vi "ErrorHandler.vi"(8 "error in (no error)":errorcluster, 11 "queue in":refnum<queue>) -> (0 "error out":errorcluster)   [LabVIEW 2024]
uses:
  Controls/MainStates.ctl
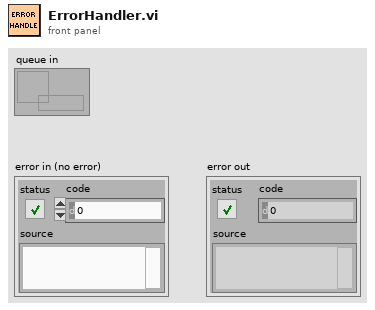
[diagram p1: front panel]
types:
  T1 = typedef "MainStates.ctl" = enum16{"Init", "Get Path", "Get Files", "Set Extension", "Check for Dups", "Clean", "Add Prefix", "Replace", "Periods", "Strip Prefix", "Commit", "Wait for Input", "Exit"}
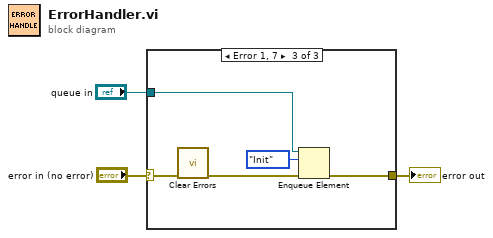
[diagram p0: block diagram]
diagram:
  n1 = case shown="Error 1, 7" "error in (no error)" {
    selector: "error in (no error)" -> [w4 w5 w10]
    tunnel: [w4 w5 w8] -> w2
    tunnel: "queue in" -> [_ _ w7]
    frame No Error {
    }
    frame Default {
    }
    frame Error {
      n2 = call <vilib>:"Clear Errors.vi"("error in (no error)"=w10) -> ("error out"=w9:errorcluster)  [unwired: 5 in, 1 out]
      n3 = Enqueue Element(queue=w7, element=MainStates."Init", error in (no error)=w9) -> (error out=w8:errorcluster)  [unwired: 1 in, 2 out]
    }
  }
  "error out" <- w2
